vi "Asylum_ReadString.vi"(8 "error in (no error)":errorcluster, 10 "parameterName":string, 11 "Application":refnum<k7>) -> (0 "error out":errorcluster, 2 "results":string, 3 "Application":refnum<k7>)   [LabVIEW 2020]
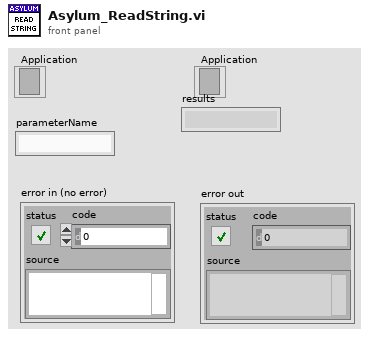
[diagram p1: front panel]
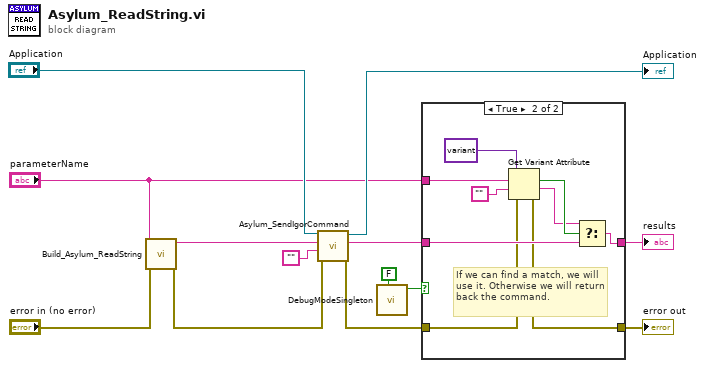
[diagram p0: block diagram]
diagram:
  n1 = call "Build_Asylum_ReadString.vi"("error in (no error)"="error in (no error)", "parameterName"="parameterName") -> ("error out"=w10:errorcluster, "String"=w12:string)  [unwired: 8 in]
  n2 = call "Asylum_SendIgorCommand.vi"("error in (no error)"=w10, "Format"="", "command"=w12, "Application In"="Application") -> ("error out"=w7:errorcluster, "results"=w4:string, "Application Out"=→"Application":refnum<k7>)  [unwired: 4 in, 1 out]
  n3 = call "DebugModeSingleton.vi"("Write?"=FALSE) -> ("Debug Mode?"=w3:bool)  [unwired: 10 in]
  n4 = case shown="True" w3 {
    tunnel: w7 -> [w14 w16]
    tunnel: [w14 w17] -> w6
    tunnel: [w15 w19] -> w5
    tunnel: w4 -> [w15 w18]
    tunnel: "parameterName" -> [_ w23]
    frame False {
    }
    frame True {
      # "If we can find a match, we will use it. Otherwise we will return back the command."
      n5 = Get Variant Attribute(Variant=variant variant ("Notes LUT"), name=w23, default value (empty Variant)="", error in=w16) -> (names=w21:bool, values=w20:string, error out=w17:errorcluster)  [unwired: 1 out]
      n6 = Select(t=w20, s=w21, f=w18) -> (s? t:f=w19:string)
    }
  }
  "error out" <- w6
  "results" <- w5
